vi "IniToken SupportedList.vi"() -> (3 "Array":T1[](array[typedef]))   [LabVIEW 2020]
uses:
  Def-IniTokenCluster.ctl
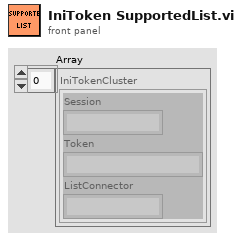
[diagram p1: front panel]
types:
  T1 = typedef "Def-IniTokenCluster.ctl" = cluster{"Session":string, "Token":string, "ListConnector":string}
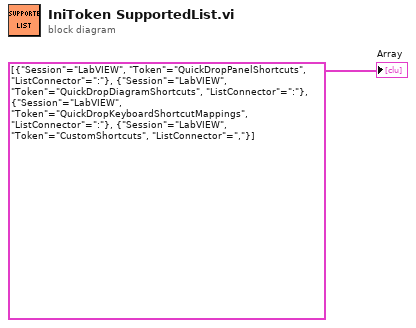
[diagram p0: block diagram]
diagram:
  "Array" <- T1[] [{"Session"="LabVIEW", "Token"="QuickDropPanelShortcuts", "ListConnector"=":"}, {"Session"="LabVIEW", "Token"="QuickDropDiagramShortcuts", "ListConnector"=":"}, {"Session"="LabVIEW", "Token"="QuickDropKeyboardShortcutMappings", "ListConnector"=":"}, {"Session"="LabVIEW", "Token"="CustomShortcuts", "ListConnector"=","}] ("Array")
